vi "Loop Computation.vi"(2 "Array Params":dbl[](array[numeric]), 3 "Array x":dbl[](array[numeric]), 4 "y key":u16, 5 "x key":u16) -> (0 "Array y":dbl[](array[numeric]), 1 "Array Output Params":dbl[](array[numeric]))   [LabVIEW 2020]
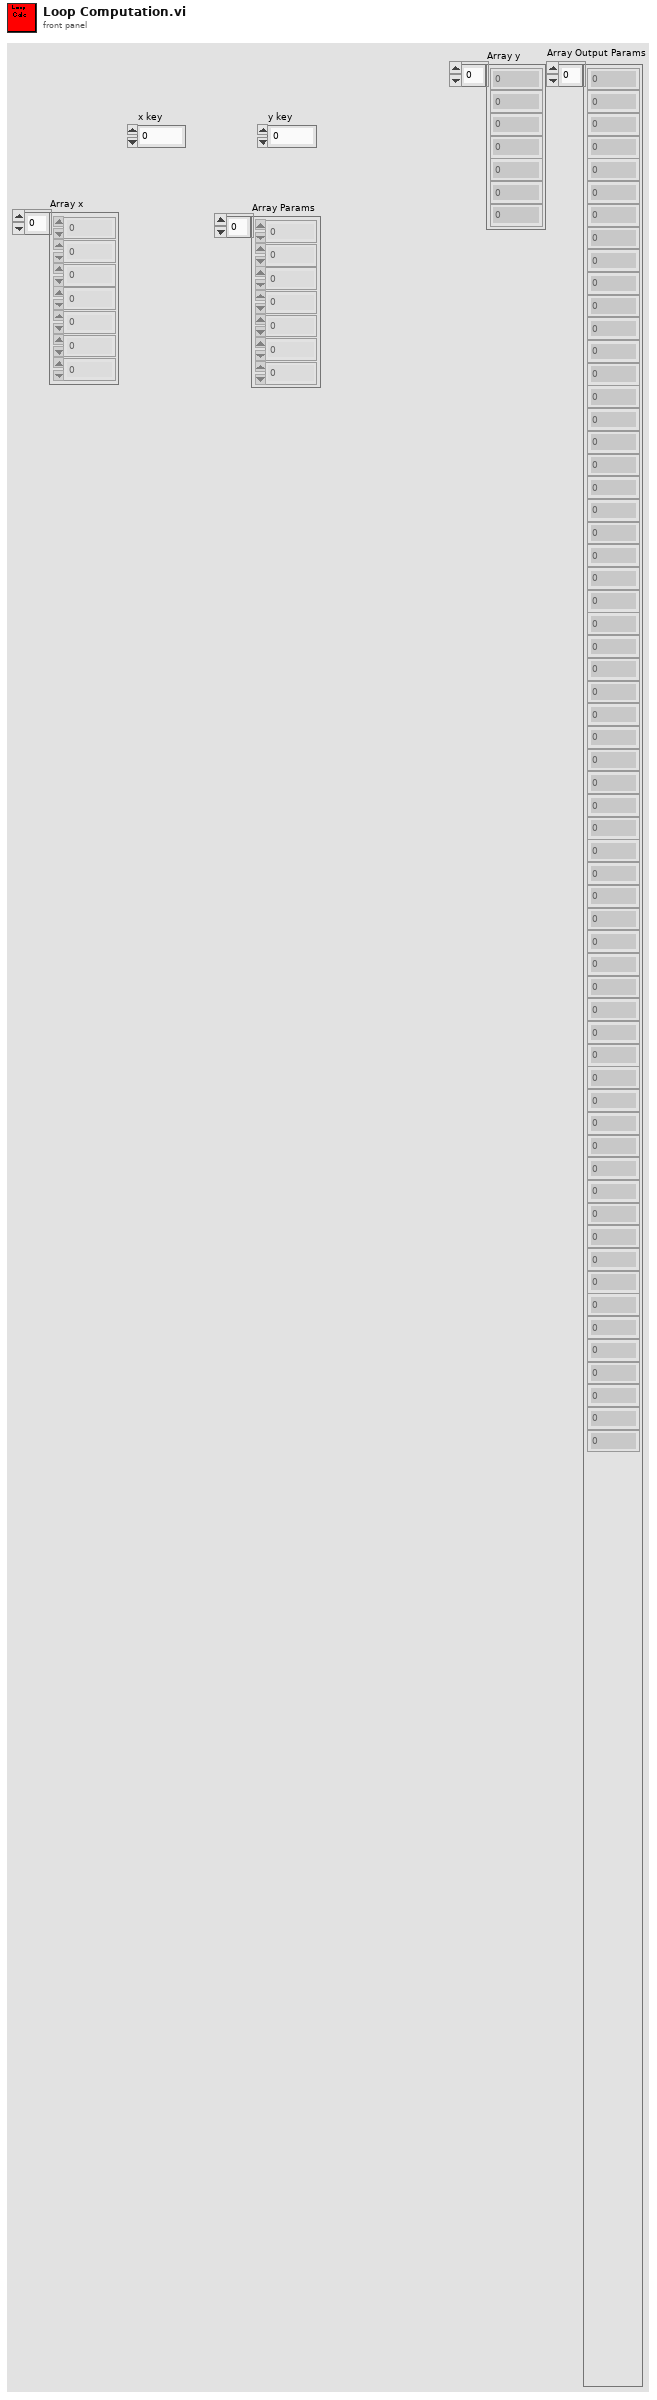
[diagram p1: front panel]
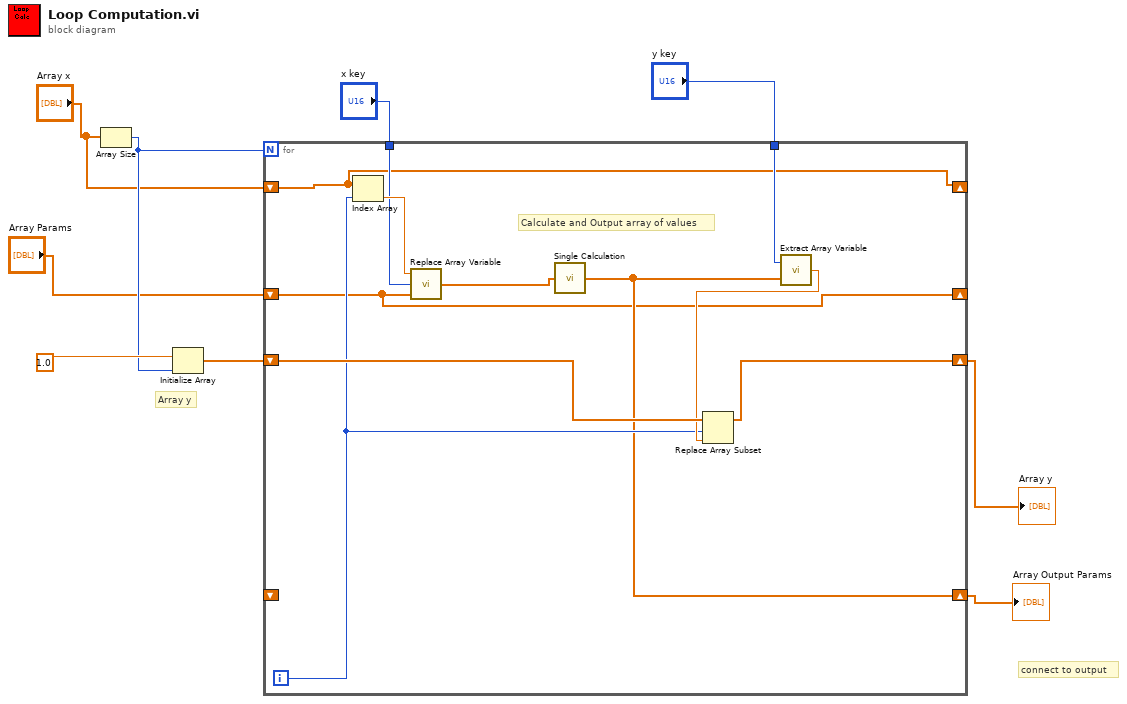
[diagram p0: block diagram]
diagram:
  # "connect to output"
  # "Array y"
  n1 = Array Size(array="Array x") -> (size(s)=w8:i32)
  n2 = Initialize Array(1.0, w8) -> (w3:dbl[])
  n3 = for {
    N: w8 -> [_]
    shift-right: [w10] -> _
    shift-left: "Array x" -> [w10]
    tunnel: "x key" -> [w19]
    shift-right: [w11] -> _
    shift-left: "Array Params" -> [w11]
    tunnel: "y key" -> [w18]
    shift-right: [w16] -> w2
    shift-left: w3 -> [w17]
    shift-right: [w12] -> w1
    shift-left: _ -> [_]
    i -> [w14]
    # "Calculate and Output array of values"
    n4 = Index Array(array=w10, index=w14) -> (element=w20:dbl)
    n5 = call "Replace Array Variable.vi"("In array"=w11, "Cluster Key"=w19, "New x Value"=w20) -> ("Out Array"=w13:dbl[])
    n6 = call "Single Calculation.vi"("Array Input"=w13) -> ("Array Output"=w12:dbl[])
    n7 = call "Extract Array Variable.vi"("In array"=w12, "Cluster Key"=w18) -> ("Out Variable"=w15:dbl)
    n8 = Replace Array Subset(array=w17, new element=w15, index=w14) -> (w16:dbl[])
  }
  "Array y" <- w2
  "Array Output Params" <- w1
